vi "Set Column Widths.vi"(9 "widest value strings":string[](array[string]), 10 "column headers":string[](array[string]), 11 "MulticolumnListbox in":refnum<vi>) -> (3 "MulticolumnListbox out":refnum<vi>)   [LabVIEW 2018, in "NI_TDMS File Viewer.lvlib"]
uses:
  NI_TDMS File Viewer.lvlib
  <vilib>/Utility/miscctls.llb/LVRowAndColumnTypeDef.ctl
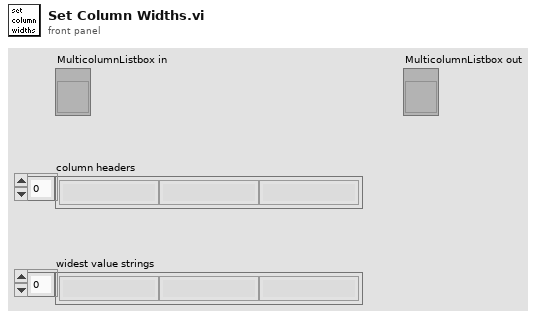
[diagram p1: front panel]
types:
  T1 = enum16{"User-specified Font", "Application Font", "System Font", "Dialog Font"}
  T2 = typedef "LVRowAndColumnTypeDef.ctl" = cluster{"Row":i32, "Column":i32}
  T3 = cluster{"left":i16, "top":i16, "right":i16, "bottom":i16}
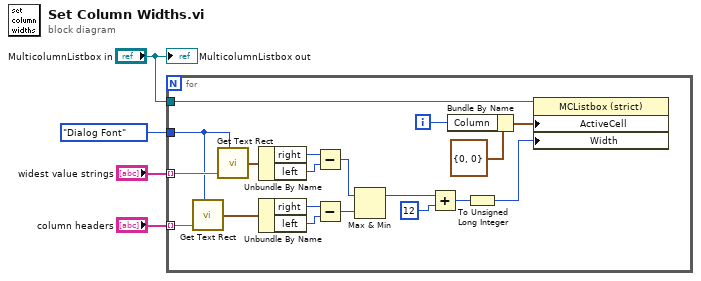
[diagram p0: block diagram]
diagram:
  n1 = for {
    tunnel: "widest value strings" -> [w18] mode=indexing
    tunnel: "column headers" -> [w14] mode=indexing
    tunnel: T1."Dialog Font" ("desired font(Application)") -> [w9]
    tunnel: "MulticolumnListbox in" -> [w5]
    i -> [w22]
    n2 = call <vilib>:"Get Text Rect.vi"("desired font(Application)"=w9, "text"=w14) -> ("rect"=w15:T3)  [unwired: 7 in]
    n3 = call <vilib>:"Get Text Rect.vi"("desired font(Application)"=w9, "text"=w18) -> ("rect"=w21:T3)  [unwired: 7 in]
    n4 = Unbundle By Name(w21) -> ("right"=w19:i16, "left"=w20:i16)
    n5 = Unbundle By Name(w15) -> ("right"=w17:i16, "left"=w16:i16)
    n6 = Subtract(x=w19, y=w20) -> (x-y=w13:i16)
    n7 = Subtract(x=w17, y=w16) -> (x-y=w12:i16)
    n8 = Max & Min(x=w13, y=w12) -> (max(x,y)=w11:i16)  [unwired: 1 out]
    n9 = Add(x=w11, y=i16 12) -> (x+y=w7:i16)
    n10 = Bundle By Name(cluster=T2 {"Row"=0, "Column"=0} ("Active Cell:Active Cell"), "Column"=w22) -> (w23:T2)
    n11 = To Unsigned Long Integer(number=w7) -> (unsigned 32bit integer=w6:u32)
    n12 = property on="Property Node" class="MCListbox (strict)"(reference=w5, "ActiveCell"=w23, "Width"=w6) -> ()  [unwired: 1 in, 2 out]
  }
  "MulticolumnListbox out" <- "MulticolumnListbox in"
